vi "Camera Finder.vi"() -> (2 "Image type":T1[](array[typedef]) items=["Grayscale (U8)", "Grayscale (I16)", "Grayscale (SGL)", "Complex (CSG)", "RGB (U32)", "HSL (U32)", "RGB (U64)", "Grayscale (U16)"], 3 "IMAQ Interfaces":string[](array[string]))   [LabVIEW 2014]
uses:
  <vilib>/vision/driver/NI_Vision_Acquisition_Software.lvlib
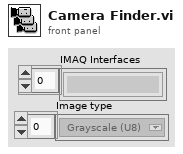
[diagram p1: front panel]
types:
  T1 = typedef "Image Type" = u32
  T2 = typedef "IMAQ Image.ctl" = refnum<image>
  T3 = cluster{"Type":u32, "Version":u32, "Flags":u32, "SerialNumberHigh":u32, "SerialNumberLow":u32, "BusType":u32, "InterfaceName":string, "VendorName":string, "ModelName":string, "CameraFileName":string, "CameraAttributeURL":string}[]
  T4 = typedef "IMAQdx.ctl" = refnum<k21>
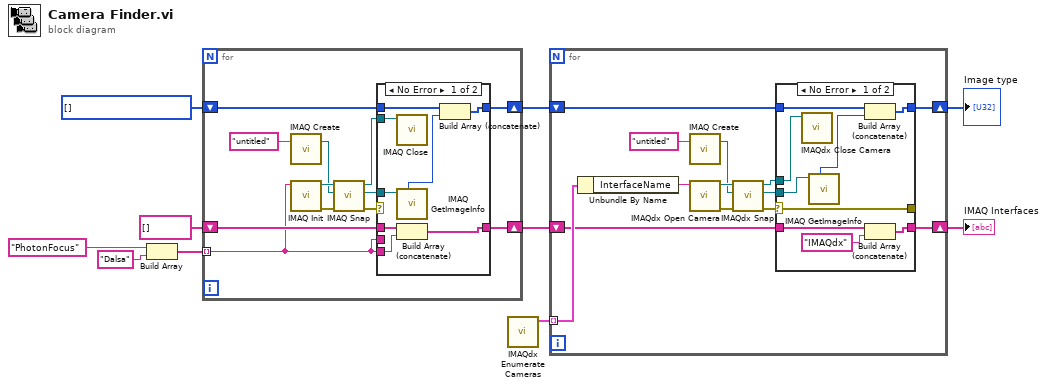
[diagram p0: block diagram]
diagram:
  w6 = T1[] [] items=["Grayscale (U8)", "Grayscale (I16)", "Grayscale (SGL)", "Complex (CSG)", "RGB (U32)", "HSL (U32)", "RGB (U64)", "Grayscale (U16)"] ("Array")
  n1 = Build Array("PhotonFocus", "Dalsa") -> (w9:string[])
  n2 = for {
    tunnel: w9 -> [w14] mode=indexing
    shift-right: [w13] -> w4
    shift-left: string[] [] -> [w15]
    shift-right: [w11] -> w5
    shift-left: w6 -> [w12]
    n3 = call "IMAQ Create"("Image Name"="untitled") -> ("New Image"=w17:T2)  [unwired: 3 in, 2 out]
    n4 = call <vilib>:"IMAQ Init.vi"("Interface Name"=w14) -> ("error out"=w20:errorcluster, "IMAQ Session Out"=w22:refnum<k11>)  [unwired: 9 in]
    n5 = call <vilib>:"IMAQ Snap.vi"("error in (no error)"=w20, "Image In"=w17, "IMAQ Session In"=w22) -> ("error out"=w18:errorcluster, "Image Out"=w16:T2, "IMAQ Session Out"=w21:refnum<k11>)  [unwired: 6 in]
    n6 = case shown="No Error" w18 {
      tunnel: w21 -> [w30 _]
      tunnel: w14 -> [_ _]
      tunnel: w16 -> [w23 _]
      tunnel: w15 -> [w29 w31]
      tunnel: w14 -> [w28 _]
      tunnel: [w27 w31] -> w13
      tunnel: w12 -> [w26 w32]
      tunnel: [w24 w32] -> w11
      frame No Error {
        n7 = call <vilib>:"IMAQ Close.vi"("IMAQ Session In"=w30) -> ()  [unwired: 10 in, 1 out]
        n8 = call "IMAQ GetImageInfo"("Image"=w23) -> ("Image Type"=w25:T1)  [unwired: 3 in, 7 out]
        n9 = Build Array (concatenate)(w29, w28) -> (w27:string[])
        n10 = Build Array (concatenate)(w26, w25) -> (w24:T1[])
      }
      frame Error {
      }
    }
  }
  n11 = call <vilib>:"IMAQdx Enumerate Cameras.vi"() -> ("Camera Information Array"=w1:T3)  [unwired: 10 in, 1 out]
  n12 = for {
    shift-right: [w39] -> w3
    shift-left: w4 -> [w40]
    shift-right: [w41] -> w2
    shift-left: w5 -> [w42]
    tunnel: w1 -> [w44] mode=indexing
    n13 = Unbundle By Name(w44) -> ("InterfaceName"=w43:string)
    n14 = call "IMAQ Create"("Image Name"="untitled") -> ("New Image"=w37:T2)  [unwired: 3 in, 2 out]
    n15 = call <vilib>:"IMAQdx Open Camera.vi"("Session In"=w43) -> ("error out"=w34:errorcluster, "Session Out"=w38:T4)  [unwired: 9 in]
    n16 = call <vilib>:"IMAQdx Snap.vi"("error in"=w34, "Image In"=w37, "Session In"=w38) -> ("error out"=w33:errorcluster, "Image Out"=w35:T2, "Session Out"=w36:T4)  [unwired: 6 in]
    n17 = case shown="No Error" w33 {
      selector: w33 -> [w54 w57]
      tunnel: [w54 w57] -> _
      tunnel: w35 -> [w52 _]
      tunnel: w36 -> [w53 _]
      tunnel: w42 -> [w51 w56]
      tunnel: [w49 w56] -> w41
      tunnel: w40 -> [w47 w55]
      tunnel: [w46 w55] -> w39
      frame No Error {
        n18 = call <vilib>:"IMAQdx Close Camera.vi"("Session In"=w53) -> ()  [unwired: 10 in, 1 out]
        n19 = call "IMAQ GetImageInfo"("Image"=w52) -> ("Image Type"=w50:T1)  [unwired: 3 in, 7 out]
        n20 = Build Array (concatenate)(w51, w50) -> (w49:T1[])
        n21 = Build Array (concatenate)(w47, "IMAQdx") -> (w46:string[])
      }
      frame Error {
      }
    }
  }
  "IMAQ Interfaces" <- w3
  "Image type" <- w2
